vi "Comments text out.vi"(4 "comment string":string) -> (0 "Command text":string[][](array[string]))   [LabVIEW 2019]
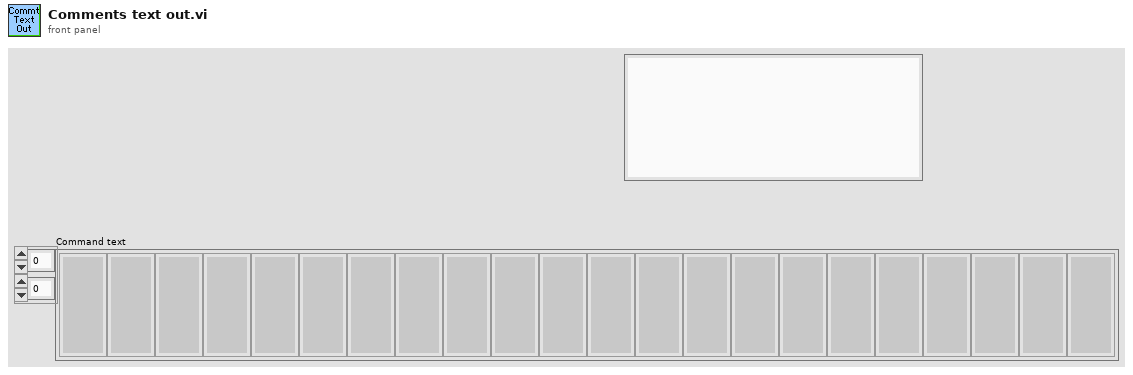
[diagram p1: front panel]
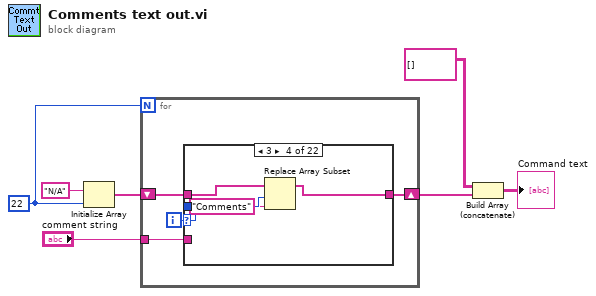
[diagram p0: block diagram]
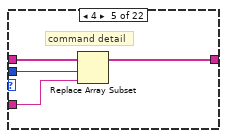
[diagram p5: hidden frame]
diagram:
  w1 = 22
  n1 = Initialize Array("N/A", w1) -> (w2:string[])
  n2 = for {
    N: w1 -> [_]
    shift-right: [w9] -> w4
    shift-left: w2 -> [w10]
    tunnel: "comment string" -> [w8]
    i -> [w11]
    n3 = case shown="3" w11 {
      tunnel: w11 -> [_ _ _ w16 w22 _ _ _ _ _ _ _ _ _ _ _ _ _ _ _ _ w42]
      tunnel: w10 -> [w12 w13 w14 w18 w19 w23 w24 w25 w26 w27 w28 w29 w30 w31 w32 w33 w34 w35 w36 w37 w38 w41]
      tunnel: [w12 w13 w14 w17 w20 w23 w24 w25 w26 w27 w28 w29 w30 w31 w32 w33 w34 w35 w36 w37 w38 w40] -> w9
      tunnel: w8 -> [_ _ _ _ w21 _ _ _ _ _ _ _ _ _ _ _ _ _ _ _ _ w39]
      frame 0, Default {
        # "Line #"
      }
      frame 1 {
      }
      frame 2 {
        # "instrument address"
      }
      frame 3 {
        n4 = Replace Array Subset(array=w18, new element="Comments" ("new element/subarray"), index=w16) -> (w17:string[])
      }
      frame 4 {
        # "command detail"
        n5 = Replace Array Subset(array=w19, new element=w21, index=w22) -> (w20:string[])
      }
      frame 5 {
        # "in  case 1"
      }
      frame 6 {
        # "in case 2"
      }
      frame 7 {
      }
      frame 8 {
      }
      frame 9 {
      }
      frame 10 {
      }
      frame 11 {
      }
      frame 12 {
      }
      frame 13 {
      }
      frame 14 {
      }
      frame 15 {
      }
      frame 16 {
      }
      frame 17 {
      }
      frame 18 {
      }
      frame 19 {
      }
      frame 20 {
      }
      frame 21 {
        n6 = Replace Array Subset(array=w41, new element=w39, index=w42) -> (w40:string[])
      }
    }
  }
  n7 = Build Array (concatenate)(string[][] [], w4) -> (→"Command text":string[][])
